vi "Init.vi"(8 "error in (no error)":errorcluster, 11 "Kasli Writer in":refnum<class "Kasli Writer.lvclass">) -> (0 "error out":errorcluster, 3 "Kasli Writer out":refnum<class "Kasli Writer.lvclass">)   [LabVIEW 2020, in "Kasli Listener and Writer.lvlib" / "Kasli Writer.lvclass"]
uses:
  Kasli Writer.lvclass
  TALOS/TALOS_PPL.lvlibp/Internal uServices/System uServices/TCP Writer/TCP Writer/TCP Writer.lvclass
  Kasli Writer.lvclass/Kasli Writer.ctl
  TALOS/TALOS_PPL.lvlibp/Father of all uServices/Father of all uServices/Father of all uServices.lvclass
  TALOS/TALOS_PPL.lvlibp/Ancestor/Ancestor/Ancestor.lvclass
  C:/Users/aegis/Documents/CIRCUS/TALOS/TALOS_PPL.lvlibp/Ancestor/Ancestor/Ancestor.lvclass
  C:/Users/aegis/Documents/CIRCUS/TALOS/TALOS_PPL.lvlibp/Father of all uServices/Father of all uServices/Father of all uServices.lvclass
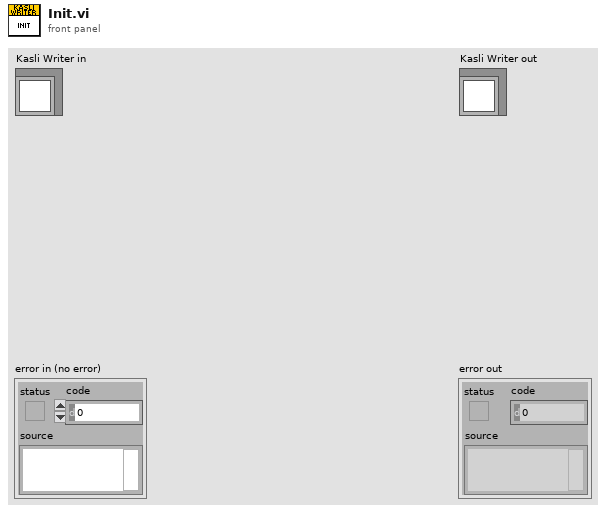
[diagram p1: front panel]
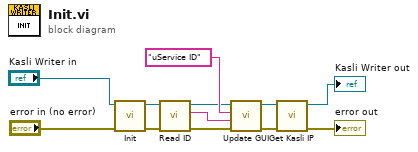
[diagram p0: block diagram]
diagram:
  n1 = call-parent "Init.vi"("error in (no error)"="error in (no error)", "TCP Writer in"="Kasli Writer in") -> ("error out"=w1:errorcluster, "TCP Writer out"=w6:refnum<class "Kasli Writer.lvclass">)  [unwired: 8 in]
  n2 = call "Read ID.vi"("error in (no error)"=w1, "Ancestor in"=w6) -> ("error out"=w8:errorcluster, "ID"=w7:string, "Ancestor out"=w4:refnum<class "Kasli Writer.lvclass">)  [unwired: 7 in]
  n3 = call "Update GUI.vi"("error in (no error)"=w8, "Data"=w7, "GUI Item Name"="uService ID", "uService Template in"=w4) -> ("error out"=w2:errorcluster, "uService Template out"=w3:refnum<class "Kasli Writer.lvclass">)  [unwired: 6 in]
  n4 = call-dynamic "Get Kasli IP.vi"("error in (no error)"=w2, "Kasli Writer in"=w3) -> ("error out"=→"error out":errorcluster, "Kasli Writer out"=→"Kasli Writer out":refnum<class "Kasli Writer.lvclass">)  [unwired: 8 in]
